vi "DriveModuleControl.vi"(4 "Outputs Enabled":bool, 6 "Pass Through Time":dbl=-1.0, 8 "error in":errorcluster, 9 "Actual State":T1={"Speed"=0.0, "Angle"={"VALUE"=0.0, "COS"=1.0, "SIN"=0.0}} {"Angle"."SIN" format="%13.4f"; "Angle"."COS" format="%13.4f"; "Angle"."VALUE" format="%13.4f"}, 10 "Desired State":T1={"Speed"=0.0, "Angle"={"VALUE"=0.0, "COS"=1.0, "SIN"=0.0}} {"Angle"."SIN" format="%13.4f"; "Angle"."COS" format="%13.4f"; "Angle"."VALUE" format="%13.4f"}, 11 "ModuleIndex":i32) -> (0 "error out":errorcluster)   [LabVIEW 2023]
uses:
  <vilib>/Rock Robotics/WPI/ThirdParty/JAS_Junk/TrajLib/Trajectory_Library.lvlib
  <vilib>/Rock Robotics/Network Tables/NT Write Number.vi
  DriveGlobal.vi
  <vilib>/Rock Robotics/WPI/ThirdParty/JAS_Junk/TrajLib/TypeDef/ROTATION2D.ctl
  <vilib>/Rock Robotics/WPI/ThirdParty/JAS_Junk/TrajLib/TypeDef/SWERVE_DRIVE_MODULE_STATE.ctl
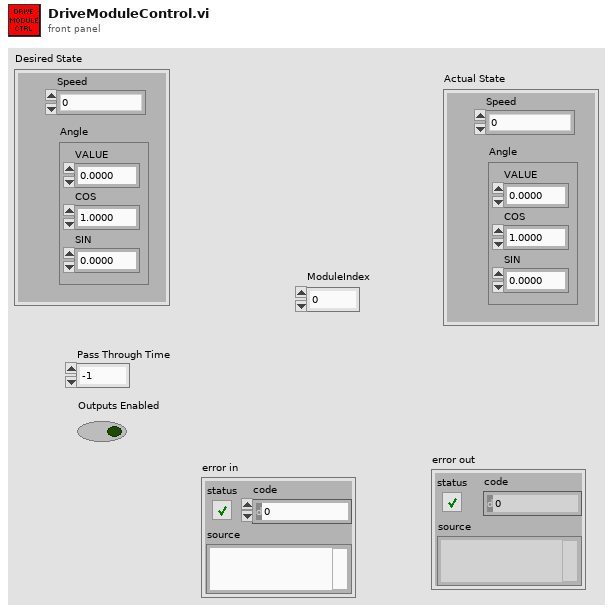
[diagram p1: front panel]
types:
  T1 = typedef "Trajectory_Library.lvlib/SWERVE_DRIVE_MODULE_STATE.ctl" = cluster{"Speed":dbl, "Angle":T2}
  T2 = typedef "Trajectory_Library.lvlib/ROTATION2D.ctl" = cluster{"VALUE":dbl, "COS":dbl, "SIN":dbl}
  T3 = typedef "WPI_MotorControlDeviceRef.ctl" = cluster{"DeviceStatus":errorcluster, "Type":T4, "PWM":cluster{"PWM Channel":T5, "DeadBand":T6}, "CAN":cluster{"Device Number":u8, "SetOutput VI Ref":variant, "GetOutput VI Ref":variant, "Enable VI Ref":variant, "Disable VI Ref":variant, "Data":variant}, "Invert":bool, "DIO PWM":cluster{"PWM \"Enable\" Channel":T5, "DIOChannel":T7, "PWM Rate":dbl}}
  T4 = typedef "WPI_MotorControlType.ctl" = enum16{"PWM", "CAN", "DIO PWM"}
  T5 = typedef "FPGA_DIOPWMChannel.ctl" = enum8{"PWM 0", "PWM 1", "PWM 2", "PWM 3", "PWM 4", "PWM 5", "PWM 6", "PWM 7", "PWM 8", "PWM 9", "PWM MXP 0", "PWM MXP 1", "PWM MXP 2", "PWM MXP 3", "PWM MXP 4", "PWM MXP 5", "PWM MXP 6", "PWM MXP 7", "PWM MXP 8", "PWM MXP 9", "Invalid"}
  T6 = typedef "WPI_PWMDeadband.ctl" = cluster{"Name":string, "maxPositivePwm":i32, "minPositivePwm":i32, "centerPwm":i32, "maxNegativePwm":i32, "minNegativePwm":i32, "angularRange":u16}
  T7 = typedef "FPGA_DIOChannel.ctl" = enum8{"DIO 0", "DIO 1", "DIO 2", "DIO 3", "DIO 4", "DIO 5", "DIO 6", "DIO 7", "DIO 8", "DIO 9", "DIO MXP 0", "DIO MXP 1", "DIO MXP 2", "DIO MXP 3", "DIO MXP 4", "DIO MXP 5", "DIO MXP 6", "DIO MXP 7", "DIO MXP 8", "DIO MXP 9", "DIO MXP 10", "DIO MXP 11", "DIO MXP 12", "DIO MXP 13", "DIO MXP 14", "DIO MXP 15", "SPI Port CS1", "SPI Port CS2", "SPI Port CS3", "SPI Port MISO", "SPI Port MOSI", "Invalid"}
  T8 = typedef "Trajectory_Library.lvlib/SIMPLE_MOTOR_FF.ctl" = cluster{"Ks":dbl, "Kv":dbl, "Ka":dbl, "KnInv":dbl}
  T9 = typedef "Trajectory_Library.lvlib/PID_ADV_LIMITS.ctl" = cluster{"MaxInput":dbl, "MinInput":dbl, "Continuous":bool, "MaxOutput":dbl, "MinOutput":dbl}
  T10 = typedef "Trajectory_Library.lvlib/PID_ADV_TUNING.ctl" = cluster{"Kf":dbl, "Kp":dbl, "Ki":dbl, "Kd":dbl, "MaximumIntegral":dbl, "MinimumIntegral":dbl, "Filter Derivative":bool, "IntegralZone":dbl}
  T11 = typedef "Trajectory_Library.lvlib/PosCtrl_Tuning_Type.ctl" = cluster{"Slope":dbl, "Offset":dbl, "Error Deadband":dbl, "At Reference Count":i32, "Negate Output":bool, "Max Allowd Position":dbl, "Min Allowd Position":dbl, "Kd":dbl, "FilterDerivative":bool}
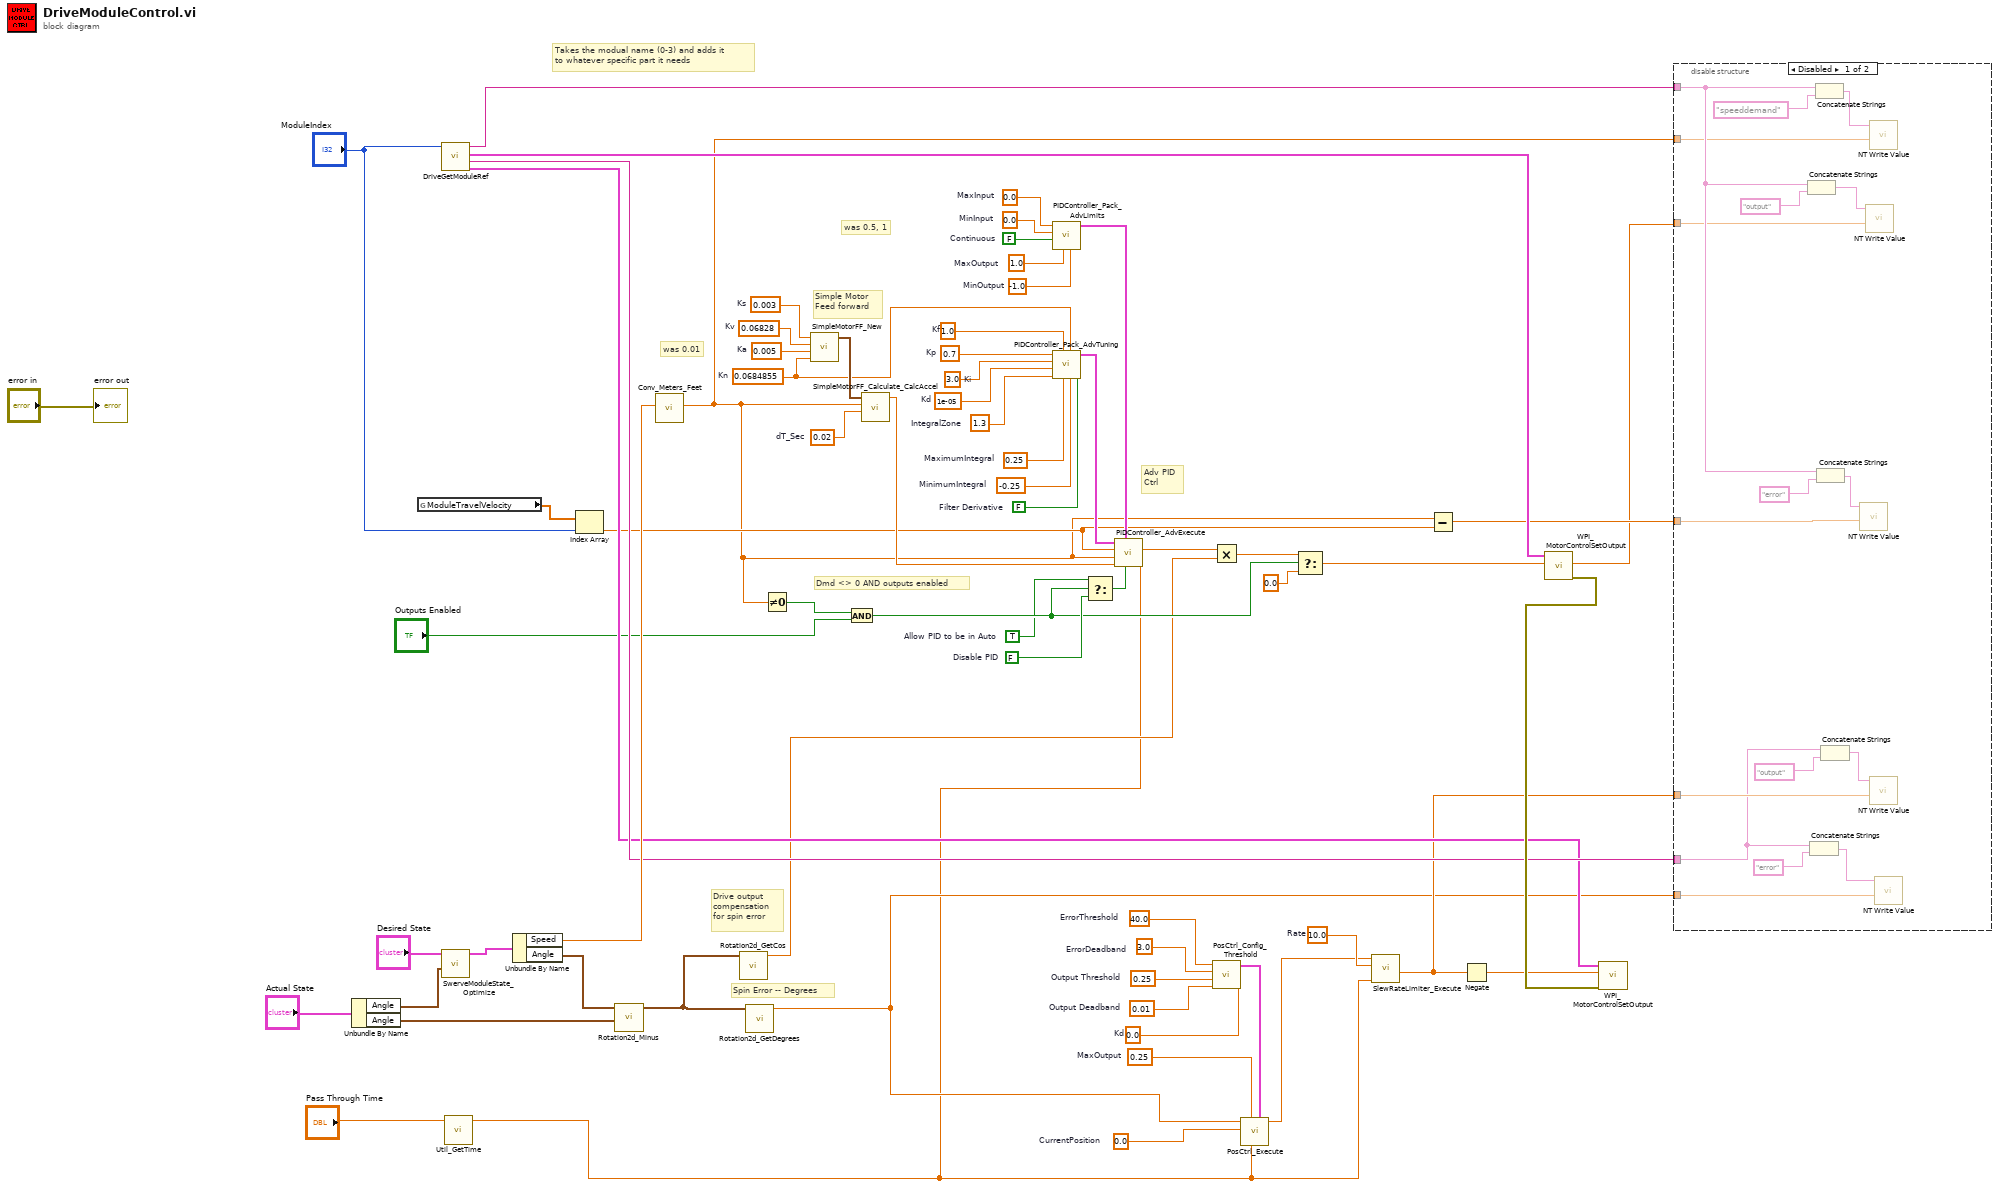
[diagram p0: block diagram]
diagram:
  w6 = 0.0  # CurrentPosition
  w13 = 0.0  # Kd
  w12 = 0.25  # MaxOutput
  w10 = 40.0  # ErrorThreshold
  w9 = 3.0  # ErrorDeadband
  w8 = 0.25  # Output Threshold
  w7 = 0.01  # Output Deadband
  w21 = 1.3  # IntegralZone
  w24 = 10.0  # Rate
  w25 = TRUE  # Allow PID to be in Auto
  w27 = FALSE  # Disable PID
  w52 = 0.7  # Kp
  w51 = 3.0  # Ki
  w50 = 1e-05  # Kd
  w49 = 1.0  # Kf
  w48 = 0.25  # MaximumIntegral
  w47 = -0.25  # MinimumIntegral
  w46 = FALSE  # Filter Derivative
  w44 = 0.0  # MinInput
  w43 = FALSE  # Continuous
  w42 = 1.0  # MaxOutput
  w45 = -1.0  # MinOutput
  w41 = 0.0  # MaxInput
  w20 = 0.0684855  # Kn
  w61 = 0.02  # dT_Sec
  w59 = 0.003  # Ks
  w58 = 0.06828  # Kv
  w57 = 0.005  # Ka
  # "Spin Error -- Degrees"
  # "Drive output\ncompensation\nfor spin error"
  # "was 0.01"
  # "was 0.5, 1"
  # "Dmd <> 0 AND outputs enabled"
  # "Adv PID\nCtrl"
  # "Simple Motor\nFeed forward"
  # "Takes the modual name (0-3) and adds it \nto whatever specific part it needs"
  n1 = Unbundle By Name("Actual State") -> ("Angle"=w64:T2, "Angle"=w22:T2)
  n2 = global read "DriveGlobal.vi" "ModuleTravelVelocity"() -> (w37:dbl[])
  n3 = call "DriveGetModuleRef.vi"("ModualNamePrefix"="ModuleIndex") -> ("SpinMot"=w53:T3, "SpinStr"=w54:string, "TravMot"=w55:T3, "TravStr"=w33:string)  [unwired: 5 in, 2 out]
  n4 = call <vilib>:"SwerveModuleState_Optimize.vi"("CurrentAngle"=w64, "Desired State"="Desired State") -> ("out SWERVE_DRIVE_MODULE_STATE"=w63:T1)  [unwired: 9 in]
  n5 = call <vilib>:"Util_GetTime.vi"("Pass_Through_Time"="Pass Through Time") -> ("FPGA_Time_Seconds"=w2:dbl)  [unwired: 8 in, 2 out]
  n6 = Unbundle By Name(w63) -> ("Speed"=w62:dbl, "Angle"=w23:T2)
  n7 = Index Array(array=w37, index="ModuleIndex") -> (element=w35:dbl)
  n8 = call <vilib>:"Rotation2d_Minus.vi"("other ROTATION"=w22, "in ROTATION"=w23) -> ("out ROTATION"=w16:T2)  [unwired: 9 in]
  n9 = call <vilib>:"Conv_Meters_Feet.vi"("Meters"=w62) -> ("Feet"=w32:dbl)  [unwired: 10 in]
  n10 = call <vilib>:"Rotation2d_GetCos.vi"("in ROTATION"=w16) -> ("Cos"=w17:dbl)  [unwired: 10 in]
  n11 = call <vilib>:"Rotation2d_GetDegrees.vi"("in ROTATION"=w16) -> ("AngleDegrees"=w5:dbl)  [unwired: 10 in]
  n12 = Not Equal To 0?(x=w32) -> (x != 0?=w29:bool)
  n13 = call <vilib>:"SimpleMotorFF_New.vi"("Kn"=w20, "Ka"=w57, "Kv"=w58, "Ks"=w59) -> ("SIMPLE_MOTOR_FF"=w60:T8)  [unwired: 7 in]
  n14 = And(x=w29, y="Outputs Enabled") -> (x .and. y?=w26:bool)
  n15 = call <vilib>:"SimpleMotorFF_Calculate_CalcAccel.vi"("dT_Sec"=w61, "VelSp"=w32, "SIMPLE_MOTOR_FF"=w60) -> ("FeedForward"=w38:dbl)  [unwired: 8 in]
  n16 = call <vilib>:"PIDController_Pack_AdvLimits.vi"("MinOutput"=w45, "MaxOutput"=w42, "Continuous"=w43, "MinInput"=w44, "MaxInput"=w41) -> ("Adv PID Limits"=w39:T9)  [unwired: 6 in]
  n17 = call <vilib>:"PIDController_Pack_AdvTuning.vi"("Filter Derivative"=w46, "MinimumIntegral"=w47, "Kn"=w20, "MaximumIntegral"=w48, "Kf"=w49, "IntegralZone"=w21, "Kd"=w50, "Ki"=w51, "Kp"=w52) -> ("Adv PID Tuning"=w40:T10)  [unwired: 2 in]
  n18 = Select(t=w25, s=w26, f=w27) -> (s? t:f=w28:bool)
  n19 = call <vilib>:"PIDController_AdvExecute.vi"("Time"=w2, "Auto"=w28, "Adv PID Limits"=w39, "FF-FeedForward"=w38, "SP-SetPoint"=w32, "PV-Measurement"=w35, "Adv PID Tuning"=w40) -> ("CO-ControlOutput"=w19:dbl)  [unwired: 2 in, 2 out]
  n20 = Multiply(x=w19, y=w17) -> (x*y=w18:dbl)
  n21 = call <vilib>:"PosCtrl_Config_Threshold.vi"("Kd"=w13, "Output Deadband"=w7, "Output Threshold"=w8, "ErrorDeadband"=w9, "ErrorThreshold"=w10) -> ("PosCtrl_Config_Params"=w11:T11)  [unwired: 5 in, 1 out]
  n22 = call <vilib>:"PosCtrl_Execute.vi"("PosCtrl_Config_Params"=w11, "Pass_Through_Time"=w2, "MaxOutput"=w12, "CurrentPosition"=w6, "TargetPosition"=w5) -> ("Output"=w4:dbl)  [unwired: 4 in, 2 out]
  n23 = Select(t=w18, s=w26, f=0.0 ("t")) -> (s? t:f=w31:dbl)
  n24 = call <vilib>:"SlewRateLimiter_Execute.vi"("Time"=w2, "PositiveRate"=w24, "Input"=w4) -> ("Output"=w14:dbl)  [unwired: 7 in, 1 out]
  n25 = Subtract(x=w32, y=w35) -> (x-y=w34:dbl)
  n26 = Negate(x=w14) -> (-x=w15:dbl)
  n27 = call <vilib>:"WPI_MotorControlSetOutput.vi"("Output"=w31, "MotorControlDevRef"=w55) -> ("error out"=w56:errorcluster)  [unwired: 7 in, 2 out]
  n28 = call <vilib>:"WPI_MotorControlSetOutput.vi"("error in (no error)"=w56, "Output"=w15, "MotorControlDevRef"=w53) -> ()  [unwired: 6 in, 3 out]
  n29 = disable-structure shown="Disabled" {
    disable-tunnel: w14 -> [w76 _]
    disable-tunnel: w54 -> [w75 _]
    disable-tunnel: w34 -> [w72 _]
    disable-tunnel: w33 -> [w71 _]
    disable-tunnel: w32 -> [w70 _]
    disable-tunnel: w31 -> [w69 _]
    disable-tunnel: w5 -> [w68 _]
    frame Disabled {
      n30 = Concatenate Strings(w71, "output" ("refnum name")) -> (w81:string)
      n31 = Concatenate Strings(w75, "error" ("refnum name")) -> (w79:string)
      n32 = Concatenate Strings(w71, "speeddemand" ("refnum name")) -> (w83:string)
      n33 = Concatenate Strings(w71, "error" ("refnum name")) -> (w73:string)
      n34 = Concatenate Strings(w75, "output" ("refnum name")) -> (w77:string)
      n35 = call-poly <vilib>:"NT Write Value.vi"("value"=w72, "name"=w73) -> ()  [unwired: 9 in, 1 out]
      n36 = call-poly <vilib>:"NT Write Value.vi"("value"=w69, "name"=w81) -> ()  [unwired: 9 in, 1 out]
      n37 = call-poly <vilib>:"NT Write Value.vi"("value"=w70, "name"=w83) -> ()  [unwired: 9 in, 1 out]
      n38 = call-poly <vilib>:"NT Write Value.vi"("value"=w76, "name"=w77) -> ()  [unwired: 9 in, 1 out]
      n39 = call-poly <vilib>:"NT Write Value.vi"("value"=w68, "name"=w79) -> ()  [unwired: 9 in, 1 out]
    }
    frame Enabled {
    }
  }
  "error out" <- "error in"
